vi "LakeShore350empty.vi"() -> ()   [LabVIEW 2015]
uses:
  SECoP.lvlib
panel:
  in  "DLL path":path=path "C:/Users/user/Desktop/x86_32"
  in  "stop":bool
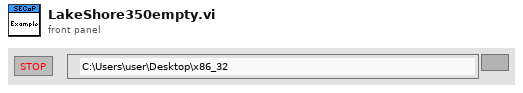
[diagram p1: front panel]
types:
  T1 = typedef "SECoP.lvlib/SECoP-libraries.ctl" = cluster{"serverDLL":path, "variantDLL":path, "cleanup_mode":bool}
  T2 = typedef "SECoP.lvlib/SECoP-action.ctl" = enum32{"any action", "read", "change", "do cmd"}
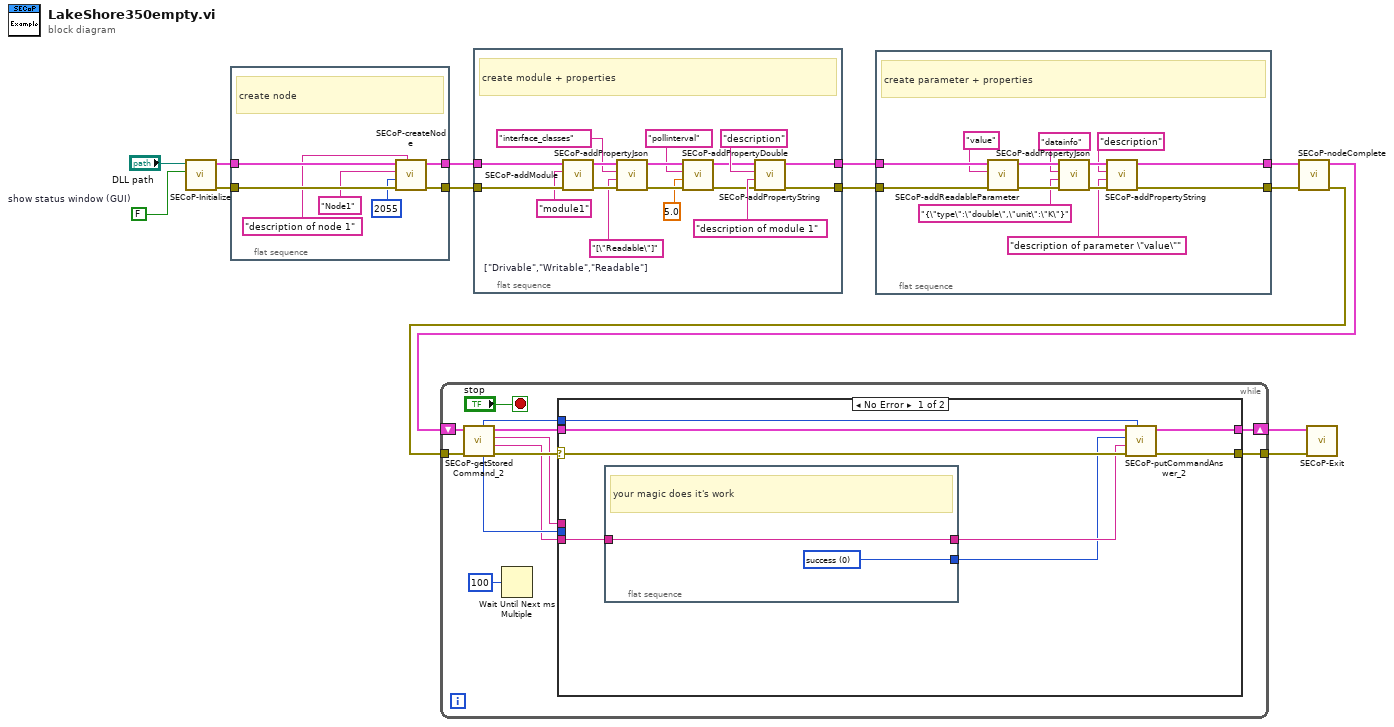
[diagram p0: block diagram]
diagram:
  w1 = FALSE  # show status window (GUI)
  n1 = call "SECoP-Initialize.vi"("show status window (GUI)"=w1, "DLL path (in)"="DLL path") -> ("error out"=w12:errorcluster, "DLL path (out)"=w13:T1)  [unwired: 8 in]
  n2 = flat-sequence {
    tunnel: w13 -> [w21]
    tunnel: w12 -> [w20]
    tunnel: [w19] -> w11
    tunnel: [w15] -> w10
    frame #0 {
      # "create node"
      n3 = call "SECoP-createNode.vi"("description"="description of node 1", "error in (no error)"=w20, "TCP port"=u16 2055, "node id"="Node1" ("id"), "DLL path (in)"=w21) -> ("error out"=w15:errorcluster, "DLL path (out)"=w19:T1)  [unwired: 5 in]
    }
  }
  n4 = flat-sequence {
    tunnel: w11 -> [w38]
    tunnel: w10 -> [w37]
    tunnel: [w31] -> w7
    tunnel: [w30] -> w6
    frame #0 {
      w32 = "[\"Readable\"]"  # ["Drivable","Writable","Readable"]
      # "create module + properties"
      n5 = call "SECoP-addModule.vi"("error in (no error)"=w37, "module name"="module1" ("name"), "DLL path (in)"=w38) -> ("error out"=w34:errorcluster, "DLL path (out)"=w35:T1)  [unwired: 7 in]
      n6 = call "SECoP-addPropertyJson.vi"("error in (no error)"=w34, "property value"=w32, "property name"="interface_classes" ("name"), "DLL path (in)"=w35) -> ("error out"=w25:errorcluster, "DLL path (out)"=w27:T1)  [unwired: 6 in]
      n7 = call "SECoP-addPropertyDouble.vi"("error in (no error)"=w25, "property value"=5.0, "property name"="pollinterval", "DLL path (in)"=w27) -> ("error out"=w24:errorcluster, "DLL path (out)"=w26:T1)  [unwired: 6 in]
      n8 = call "SECoP-addPropertyString.vi"("error in (no error)"=w24, "property value"="description of module 1" ("name"), "property name"="description" ("name"), "DLL path (in)"=w26) -> ("error out"=w30:errorcluster, "DLL path (out)"=w31:T1)  [unwired: 6 in]
    }
  }
  n9 = flat-sequence {
    tunnel: w7 -> [w51]
    tunnel: w6 -> [w50]
    tunnel: [w49] -> w3
    tunnel: [w48] -> w2
    frame #0 {
      # "create parameter + properties"
      n10 = call "SECoP-addReadableParameter.vi"("error in (no error)"=w50, "parameter name"="value", "DLL path (in)"=w51) -> ("error out"=w44:errorcluster, "DLL path (out)"=w45:T1)  [unwired: 7 in]
      n11 = call "SECoP-addPropertyJson.vi"("error in (no error)"=w44, "property value"="{\"type\":\"double\",\"unit\":\"K\"}", "property name"="datainfo" ("name"), "DLL path (in)"=w45) -> ("error out"=w46:errorcluster, "DLL path (out)"=w47:T1)  [unwired: 6 in]
      n12 = call "SECoP-addPropertyString.vi"("error in (no error)"=w46, "property value"="description of parameter \"value\"", "property name"="description" ("name"), "DLL path (in)"=w47) -> ("error out"=w48:errorcluster, "DLL path (out)"=w49:T1)  [unwired: 6 in]
    }
  }
  n13 = call "SECoP-nodeComplete.vi"("error in (no error)"=w2, "DLL path (in)"=w3) -> ("error out"=w5:errorcluster, "DLL path (out)"=w4:T1)  [unwired: 8 in]
  n14 = while {
    shift-right: [w63] -> w9
    shift-left: w4 -> [w61]
    tunnel: w5 -> [w60]
    tunnel: [w53] -> w8
    stop <- "stop" stop-if-true
    n15 = call "SECoP-getStoredCommand_2.vi"("error in (no error)"=w60, "DLL path (in)"=w61) -> ("error out"=w58:errorcluster, "arguments/setvalue"=w54:string, "command/parameter path"=w55:string, "DLL path (out)"=w59:T1, "action"=w56:T2, "command id"=w57:u64)  [unwired: 4 in]
    n16 = Wait Until Next ms Multiple(millisecond multiple=u32 100) -> ()  [unwired: 1 out]
    n17 = case shown="No Error" w58 {
      selector: w58 -> [w71 w74]
      tunnel: w59 -> [w70 w75]
      tunnel: [w69 w75] -> w63
      tunnel: w57 -> [w68 _]
      tunnel: w55 -> [_ _]
      tunnel: w54 -> [w66 _]
      tunnel: w56 -> [_ _]
      tunnel: [w67 w74] -> w53
      frame No Error {
        n18 = flat-sequence {
          tunnel: w66 -> [w73]
          tunnel: [w73] -> w65
          tunnel: [w72] -> w64
          frame #0 {
            w72 = 0 items=["warn: missing properties"=4, "warn: buffer too small"=3, "warn: custom property"=2, "warn: no description"=1, "success"=0, "error: unknown command"=-1, "error: invalid name"=-2, "error: invalid node"=-3, "error: invalid module"=-4, "error: invalid parameter"=-5, "error: invalid property"=-6, "error: invalid command"=-7, "error: not implemented"=-8, "error: readonly"=-9, "error: no data"=-10, "error: no memory"=-11, "error: not initialized"=-12, "error: invalid value"=-13, "error: missing mandatory prop"=-14, "error: no setter/getter"=-15, "error: no setter"=-16, "error: no getter"=-17, "error: name already in use"=-18] ("SECoP error")
            # "your magic does it's work"
          }
        }
        n19 = call "SECoP-putCommandAnswer_2.vi"("command id"=w68, "error in (no error)"=w71, "value"=w65, "SECoP error"=w64, "DLL path (in)"=w70) -> ("error out"=w67:errorcluster, "DLL path (out)"=w69:T1)  [unwired: 5 in]
      }
      frame Error {
      }
    }
  }
  n20 = call "SECoP-Exit.vi"("error in (no error)"=w8, "DLL path (in)"=w9) -> ()  [unwired: 9 in, 1 out]
